vi "Save Image to png.vi"(4 "Channel":string, 6 "image metadata":T2={"serial channel"=0.0, "frame number"=0, "data type"=enum."Frame Start", "width"=0, "height"=0, "image bytes"=0, "total bytes"=0, "little endian"=FALSE, "Status"="Ready for Acquisition"}, 7 "raw display notifier":refnum<notifier>, 8 "error in":errorcluster, 11 "Last displayed image data":u32[](array[numeric])) -> (0 "error out":errorcluster)   [LabVIEW 2025, in "Automotive Vision.lvclass"]
uses:
  Automotive Vision.lvclass
  Program Files/NI/LVAddons/flexrioii/1/ProjectTemplates/Source/FlexRIO/NI148X/Getting Started/Host/Common/Types/Serial Channel Display Parameters.ctl
  <vilib>/vision/Image Controls.llb/IMAQ Image.ctl
  Program Files/NI/LVAddons/flexrioii/1/ProjectTemplates/Source/FlexRIO/NI148X/Getting Started/Host/Common/Types/RAW Interpretation for Display.ctl
  <instrlib>/FlexRIO/CSI-2/v2/Common/Types/LLP Data Type.ctl
  Automotive Vision.lvclass/Automotive Vision.ctl
  Automotive-Vision OOB Data Transfer/Automotive-Vision OOB Data Transfer.lvlib
  <instrlib>/FlexRIO/Automotive Vision Utility/v1/Host/Automotive Vision Utility.lvlib
  Program Files/NI/LVAddons/flexrioii/1/ProjectTemplates/Source/FlexRIO/NI148X/Getting Started/Host/Common/GettingStarted_Common_148X_Host.lvlib
  <instrlib>/FlexRIO/CSI-2/v2/Common/NI CSI-2 API Common v2.lvlib
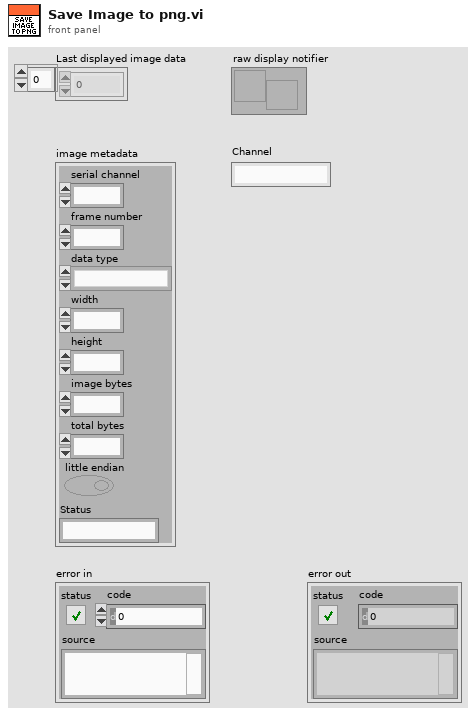
[diagram p1: front panel]
types:
  T1 = typedef "NI CSI-2 API Common v2.lvlib/LLP Data Type.ctl" = enum8{"Frame Start", "Frame End", "Line Start", "Line End", "End of Transmission", "Reserved 0", "Reserved 1", "Reserved 2", "Generic Short Packet 1", "Generic Short Packet 2", "Generic Short Packet 3", "Generic Short Packet 4", "Generic Short Packet 5", "Generic Short Packet 6", "Generic Short Packet 7", "Generic Short Packet 8", "Null", "Blanking Data", "Embedded 8-bit non Image Data", "Generic Long Packet 1", "Generic Long Packet 2", "Generic Long Packet 3", "Generic Long Packet 4", "Reserved 3", "YUV420 8-bit", "YUV420 10-bit", "Legacy YUV420 8-bit", "Reserved 4", "YUV420 8-bit Chroma Shifted", "YUV420 10-bit Chroma Shifted", "YUV422 8-bit", "YUV422 10-bit", "RGB444", "RGB555", "RGB565", "RGB666", "RGB888", "Reserved 5", "Reserved 6", "RAW 24", "RAW 6", "RAW 7", "RAW 8", "RAW 10", "RAW 12", "RAW 14", "RAW 16", "RAW 20", "User Defined 8-bit Data 1", "User Defined 8-bit Data 2", "User Defined 8-bit Data 3", "User Defined 8-bit Data 4", "User Defined 8-bit Data 5", "User Defined 8-bit Data 6", "User Defined 8-bit Data 7", "User Defined 8-bit Data 8", "USL Command", "Reserved 7", "Reserved 8", "Reserved 9", "Reserved 10", "Reserved 11", "Reserved 12", "LRTE EPD Spacer"}
  T2 = cluster{"serial channel":fxp<+,3,3>, "frame number":u16, "data type":T1, "width":u16, "height":u16, "image bytes":u32, "total bytes":u32, "little endian":bool, "Status":string}
  T3 = typedef "Automotive-Vision OOB Data Transfer.lvlib/OOB to Logic Data.ctl" = cluster{"PauseResume":bool, "ExportPath":string, "ExportType":u16, "Export":bool}
  T4 = typedef "GettingStarted_Common_148X_Host.lvlib/Serial Channel Display Parameters.ctl" = cluster{"images":cluster{"grayscale":T5, "color":T5}, "RAW parameters":cluster{"interpretation":T6, "bayer parameters":cluster{"pattern":i32, "algorithm":i32, "red gain":dbl, "green gain":dbl, "blue gain":dbl}}}
  T5 = typedef "IMAQ Image.ctl" = refnum<image>
  T6 = typedef "GettingStarted_Common_148X_Host.lvlib/RAW Interpretation for Display.ctl" = enum16{"Grayscale", "Bayer", "RGB", "YUV422", "YUV420", "Legacy YUV420"}
  T7 = cluster{"pattern":i32, "algorithm":i32, "red gain":dbl, "green gain":dbl, "blue gain":dbl}
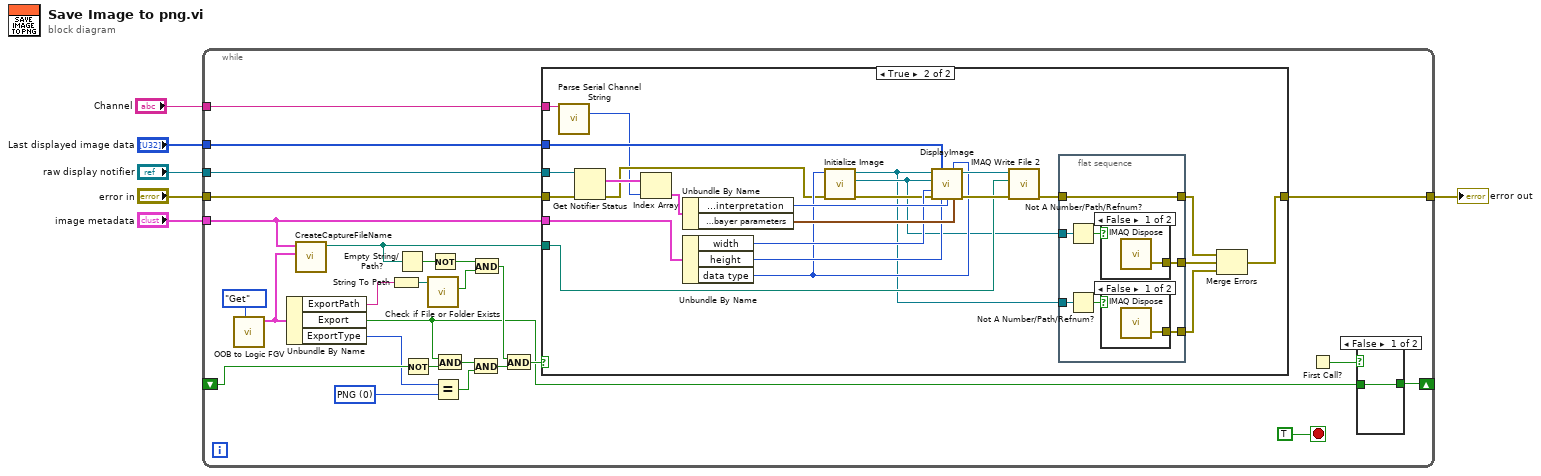
[diagram p0: block diagram]
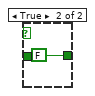
[diagram p5: hidden frame]
diagram:
  n1 = while {
    shift-right: [w30] -> _
    shift-left: _ -> [w28]
    tunnel: "Last displayed image data" -> [w24]
    tunnel: "raw display notifier" -> [w23]
    tunnel: "image metadata" -> [w22]
    tunnel: "error in" -> [w20]
    tunnel: [w19] -> w2
    tunnel: "Channel" -> [w7]
    stop <- TRUE stop-if-true
    w26 = u16 0 items=["PNG", "RAW"] ("ExportType")
    n2 = call "OOB to Logic FGV.vi"("Op (Get)"=enum16{"Get", "Set"}."Get") -> ("OOB to Logic Data out"=w21:T3)  [unwired: 9 in, 1 out]
    n3 = Unbundle By Name(w21) -> ("ExportPath"=w8:string, "Export"=w13:bool, "ExportType"=w27:u16)
    n4 = call "CreateCaptureFileName.vi"("OOB to Logic Data out"=w21, "image metadata"=w22) -> ("Path"=w15:path)  [unwired: 9 in]
    n5 = String To Path(string=w8) -> (path=w9:path)
    n6 = Empty String/Path?(string/path=w15) -> (empty?=w16:bool)
    n7 = Not(x=w28) -> (.not. x?=w29:bool)
    n8 = call <vilib>:"Check if File or Folder Exists.vi"("path"=w9) -> ("file or folder exists?"=w10:bool)  [unwired: 8 in, 2 out]
    n9 = Not(x=w16) -> (.not. x?=w11:bool)
    n10 = Equal?(x=w27, y=w26) -> (x = y?=w25:bool)
    n11 = And(x=w13, y=w29) -> (x .and. y?=w12:bool)
    n12 = And(x=w12, y=w25) -> (x .and. y?=w18:bool)
    n13 = And(x=w11, y=w10) -> (x .and. y?=w14:bool)
    n14 = And(x=w14, y=w18) -> (x .and. y?=w17:bool)
    n15 = case shown="True" w17 {
      tunnel: w24 -> [_ w56]
      tunnel: w23 -> [_ w59]
      tunnel: w22 -> [_ w52]
      tunnel: w15 -> [_ w48]
      tunnel: w20 -> [w34 w47]
      tunnel: [w34 w39] -> w19
      tunnel: w7 -> [_ w35]
      frame False {
      }
      frame True {
        n16 = call <instrlib>:"Parse Serial Channel String.vi"("serial channel string"=w35) -> ("channel number"=w36:i32)  [unwired: 13 in, 1 out]
        n17 = Get Notifier Status(notifier=w59, error in (no error)=w47) -> (current notification=w58:T4[], error out=w44:errorcluster)  [unwired: 3 out]
        n18 = Index Array(array=w58, index=w36) -> (element=w57:T4)
        n19 = Unbundle By Name(w57) -> ("RAW parameters.interpretation"=w54:T6, "RAW parameters.bayer parameters"=w55:T7)
        n20 = Unbundle By Name(w52) -> ("width"=w51:u16, "height"=w50:u16, "data type"=w46:T1)
        n21 = call "Initialize Image.vi"("error in (no error)"=w44, "data type"=w46) -> ("error out"=w45:errorcluster, "Gray Image Out"=w38:T5, "Color Image Out"=w37:T5)  [unwired: 7 in]
        n22 = call "DisplayImage.vi"("image color"=w37, "Image Pixel Data"=w56, "data type"=w46, "Image grayscale"=w38, "width"=w51, "error in (no error)"=w45, "height"=w50, "interpretation"=w54, "bayer parameters"=w55) -> ("display image"=w53:T5, "error out"=w49:errorcluster)  [unwired: 5 in]
        n23 = call-poly "IMAQ Write File 2"("error in (no error)"=w49, "File Path"=w48, "Image"=w53) -> ("error out"=w40:errorcluster)  [unwired: 7 in, 1 out]
        n24 = flat-sequence {
          tunnel: [w64] -> w43
          tunnel: [w63] -> w42
          tunnel: [w62] -> w41
          tunnel: w40 -> [w62]
          tunnel: w38 -> [w61]
          tunnel: w37 -> [w60]
          frame #0 {
            n25 = Not A Number/Path/Refnum?(number/path/refnum=w61) -> (NaN/Path/Refnum?=w65:bool)
            n26 = Not A Number/Path/Refnum?(number/path/refnum=w60) -> (NaN/Path/Refnum?=w66:bool)
            n27 = case shown="False" w65 {
              tunnel: [w67 _] -> w64
              frame False {
                n28 = call "IMAQ Dispose"() -> ("error out"=w67:errorcluster)  [unwired: 6 in]
              }
              frame True {
              }
            }
            n29 = case shown="False" w66 {
              tunnel: [w68 _] -> w63
              frame False {
                n30 = call "IMAQ Dispose"() -> ("error out"=w68:errorcluster)  [unwired: 6 in]
              }
              frame True {
              }
            }
          }
        }
        n31 = Merge Errors(w41, w43, w42) -> (w39:errorcluster)
      }
    }
    n32 = First Call?() -> (First Call?: T/F=w31:bool)
    n33 = case shown="False" w31 {
      tunnel: [w69 FALSE] -> w30
      tunnel: w13 -> [w69 _]
      frame False {
      }
      frame True {
      }
    }
  }
  "error out" <- w2
